vi "SetGain.vi"(8 "error in (no error)":errorcluster, 10 "Gain":dbl=1.0 min=1.0 max=3.9810717055349722, 11 "CameraLan in":refnum<class "CameraLan.lvclass">) -> (0 "error out":errorcluster, 3 "CameraLan out":refnum<class "CameraLan.lvclass">)   [LabVIEW 2013, in "CameraLan.lvclass"]
uses:
  CameraLan.lvclass
  CameraLan.lvclass/CameraLan.ctl
  <resource>/objmgr/imaqdx.rc
panel:
  out "Boolean":bool
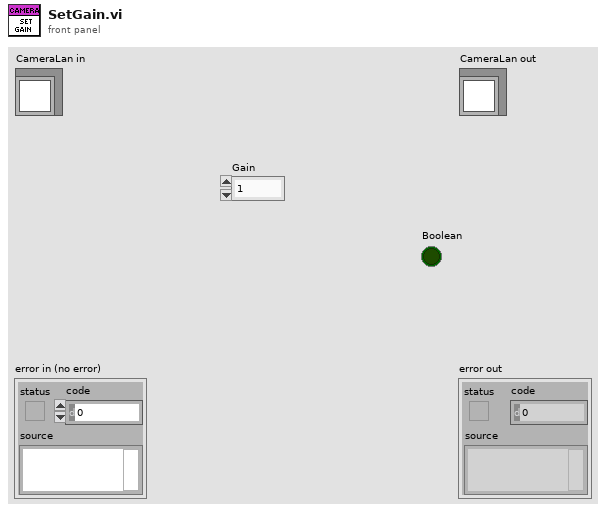
[diagram p1: front panel]
types:
  T1 = typedef "IMAQdx.ctl" = refnum<k21>
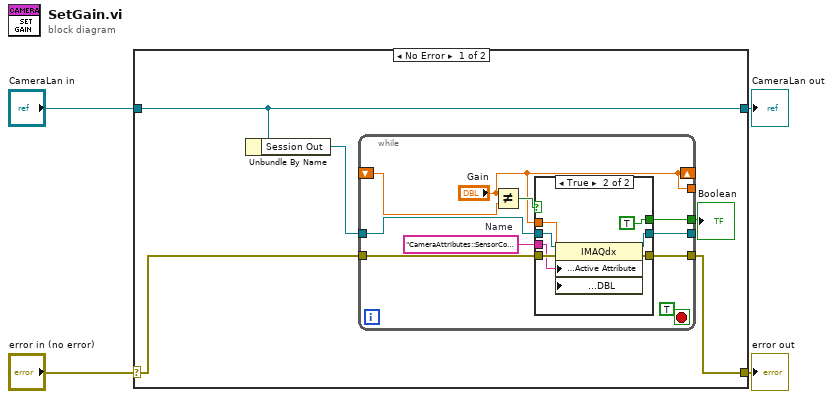
[diagram p0: block diagram]
diagram:
  n1 = case shown="No Error" "error in (no error)" {
    selector: "error in (no error)" -> [w7 w30]
    tunnel: [w6 w30] -> w3
    tunnel: [w9 w29] -> w1
    tunnel: "CameraLan in" -> [w9 w29]
    frame No Error {
      n2 = Unbundle By Name(w9) -> ("Session Out"=w8:T1)
      n3 = while {
        tunnel: w7 -> [w19]
        tunnel: [w18] -> _
        tunnel: w8 -> [w17]
        tunnel: [w16] -> w6
        shift-right: ["Gain"] -> _
        shift-left: _ -> [w13]
        tunnel: ["Gain"] -> _
        tunnel: [w10] -> w5
        stop <- TRUE stop-if-true
        w15 = "CameraAttributes::SensorControl::GainAbs"  # Name
        n4 = Not Equal?(x="Gain", y=w13) -> (x != y?=w12:bool)
        n5 = case shown="True" w12 {
          tunnel: w19 -> [w20 w28]
          tunnel: [w21 w27] -> w18
          tunnel: w17 -> [w21 w26]
          tunnel: [w20 w25] -> w16
          tunnel: w15 -> [_ w24]
          tunnel: "Gain" -> [_ w23]
          tunnel: [_ TRUE] -> w10
          frame False {
          }
          frame True {
            n6 = property class="IMAQdx"(reference=w26, error in=w28, "Camera Attributes:Active Attribute"=w24, "Camera Attributes:Value:DBL"=w23) -> (reference out=w27:T1, error out=w25:errorcluster)
          }
        }
      }
      "Boolean" <- w5
    }
    frame Error {
    }
  }
  "error out" <- w3
  "CameraLan out" <- w1
